vi "Write Step requesting configuration.vi"(8 "error in (no error)":errorcluster, 10 "Step requesting configuration":string, 11 "HW Configuration in":refnum<class "HW Configuration.lvclass">) -> (0 "error out":errorcluster, 3 "HW Configuration out":refnum<class "HW Configuration.lvclass">)   [LabVIEW 2017, in "Hardware.lvlib" / "HW Configuration.lvclass"]
uses:
  HW Configuration.lvclass
  HW Configuration.lvclass/HW Configuration.ctl
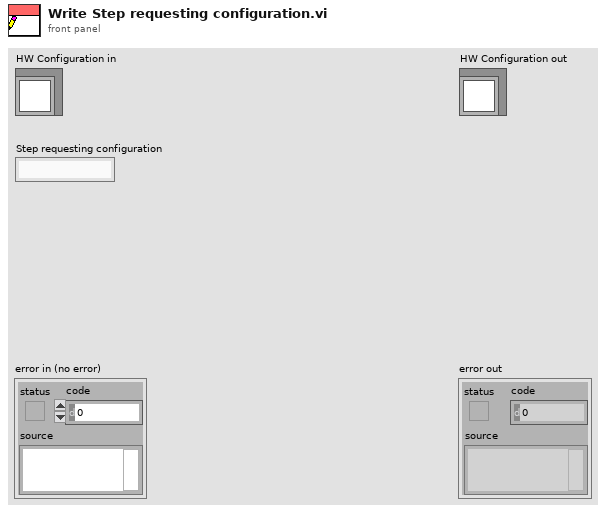
[diagram p1: front panel]
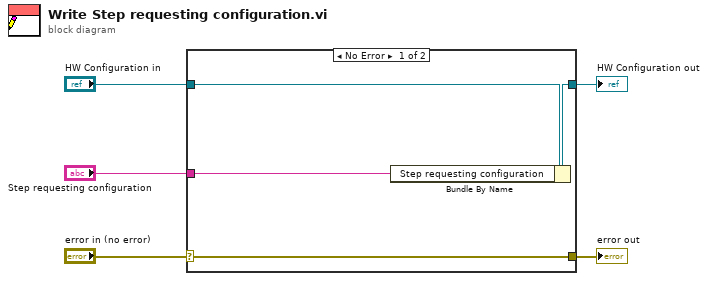
[diagram p0: block diagram]
diagram:
  n1 = case shown="No Error" "error in (no error)" {
    selector: "error in (no error)" -> [w9 w10]
    tunnel: [w9 w10] -> w4
    tunnel: [w7 w11] -> w2
    tunnel: "HW Configuration in" -> [w8 w11]
    tunnel: "Step requesting configuration" -> [w6 _]
    frame No Error {
      n2 = Bundle By Name(cluster=w8, "Step requesting configuration"=w6) -> (w7:refnum<class "HW Configuration.lvclass">)
    }
    frame Error {
    }
  }
  "error out" <- w4
  "HW Configuration out" <- w2
